vi "A33ConfigureSquare_py.vi"(8 "error in (no error)":errorcluster, 9 "Duty cycle (50%)":dbl=50.0 format="%#_12g", 10 "Channel (1: Channel1)":i32(ring)=1 items=["Channel1"=1, "Channel2"=2]) -> (0 "error out":errorcluster)   [LabVIEW 2022 SP3]
doc: "Selects the waveform shape, frequency, amplitude, offset, and phase for a standard waveform."
uses:
  <vilib>/addons/zeromq/zmq_socket.lvclass
panel:
  out "Standalone 2":bool
  out "socket out 2":refnum<class "zmq_socket.lvclass">
  in  "socket in 2":refnum<class "zmq_socket.lvclass">
  out "resulting string 2":string
  in  "Instrument 2":string="AG33600A_Gen1"
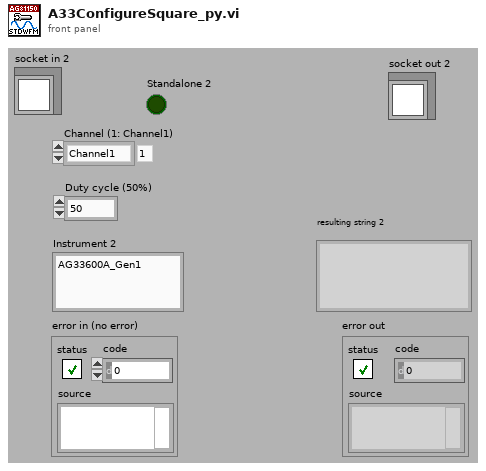
[diagram p1: front panel]
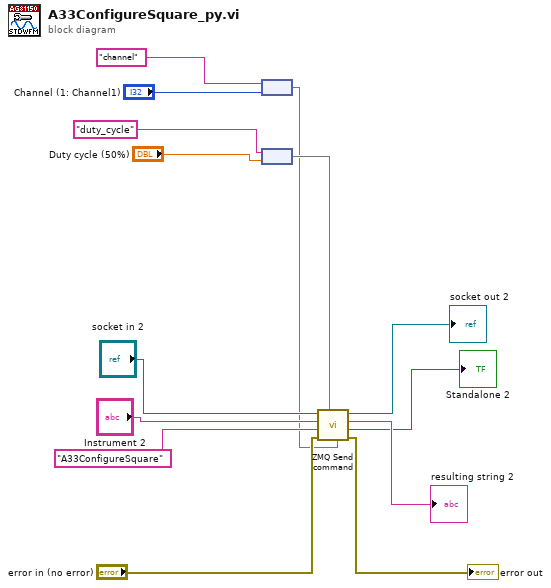
[diagram p0: block diagram]
diagram:
  n1 = node("channel" ("key"), "Channel (1: Channel1)") -> (w1:map{string, i32})
  n2 = node("duty_cycle" ("key"), "Duty cycle (50%)") -> (w2:map{string, dbl})
  n3 = call "ZMQ Send command.vi"("Int args"=w1, "DBL args"=w2, "error in"="error in (no error)", "Command"="A33ConfigureSquare", "Instrument"="Instrument 2", "socket in"="socket in 2") -> ("error out"=→"error out":errorcluster, "Standalone"=→"Standalone 2":bool, "Recieved message"=→"resulting string 2":string, "socket out"=→"socket out 2":refnum<class "zmq_socket.lvclass">)  [unwired: 2 in]
